vi "Is_TopLevel.vi"(8 "error in (no error)":errorcluster, 11 "AB_Source_RESTfulVI in":refnum<class "AB_Source_RESTfulVI.lvclass">) -> (0 "error out":errorcluster, 1 "openVIreference":bool, 2 "path":path, 3 "AB_Source_RESTfulVI out":refnum<class "AB_Source_RESTfulVI.lvclass">, 5 "readLinker":bool)   [LabVIEW 2020, in "AB_Source_RESTfulVI.lvclass"]
uses:
  <vilib>/AppBuilder/AB_Classes/Source/RESTfulVI/AB_Source_RESTfulVI.lvclass
  e:/builds/penguin/labview/branches/2020/dev/dist/vi.lib/AppBuilder/AB_Classes/Source/AB_Source.lvclass
  e:/builds/penguin/labview/branches/2020/dev/dist/vi.lib/AppBuilder/AB_Classes/Source/VI/AB_Source_VI.lvclass
  <resource>/Framework/Providers/Common/provcom_StringGlobals.vi
  <vilib>/AppBuilder/AB_Classes/Source/VI/AB_Source_VI.lvclass
  <vilib>/AppBuilder/AB_Classes/Source/AB_Source.lvclass
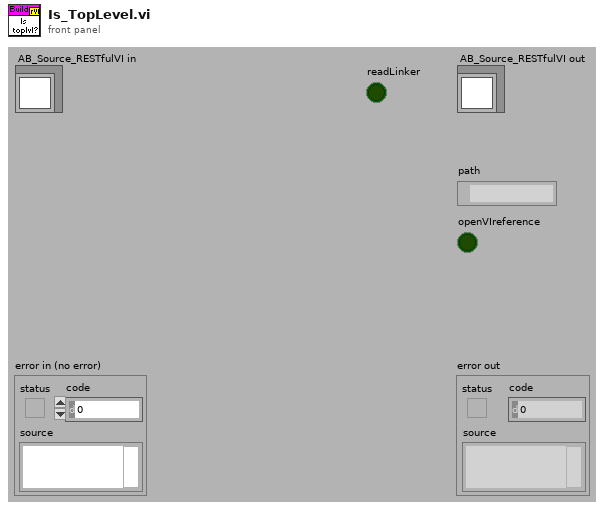
[diagram p1: front panel]
types:
  T1 = typedef "AB_Source.ctl" = cluster{"path":path, "itemID":string, "parentIndex":i32, "sourceInclusion":T2, "destinationIndex":i32, "properties":T3[], "newName":string, "lvfile":bool, "valid":bool, "eng_inBuild":bool, "eng_isNonVILink":bool, "Amalgamation":bool, "Amalgamation Piece":bool, "eng_delimitedName":string, "preventRename":bool}
  T2 = typedef "AB_Source_Inclusion.ctl" = enum16{"IncludeIfReferenced", "Include", "Exclude", "TopLevel"}
  T3 = typedef "AB_Source_Properties.ctl" = cluster{"sourcePropertyType":T4, "value":variant}
  T4 = typedef "AB_Source_Property_Type.ctl" = enum16{"Remove block diagram", "Remove front panel", "Password", "Window has title bar", "Show menu bar", "Show vertical scroll bar", "Show horizontal scroll bar", "Show toolbar", "Show Abort button", "Show fp when called", "Window behavior", "Allow user to close window", "Window run-time position", "Run when opened", "Allow debugging", "Auto error handling", "Generate guard code", "Use stack variables", "Expression folding", "Integer only", "Inline subVI"}
  T5 = typedef "AB_Source_VI.ctl" = cluster{"standardVI":bool, "dynamicDispatch":bool, "LLBtopLevel":bool, "privateDataControl":bool, "eng_hasNonVILinks":bool, "eng_reference":refnum<vi>, "eng_saveLevel":u32}
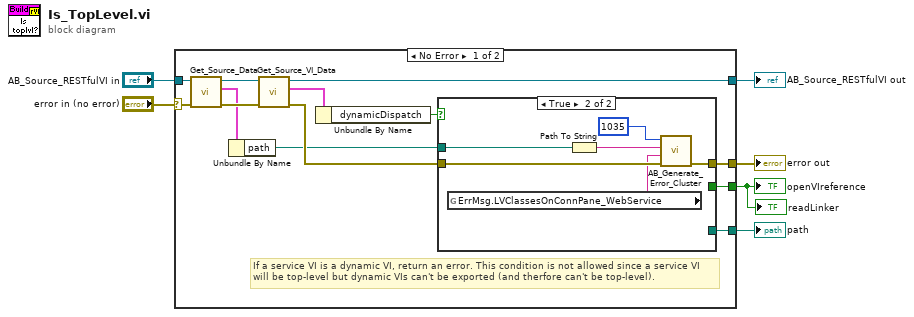
[diagram p0: block diagram]
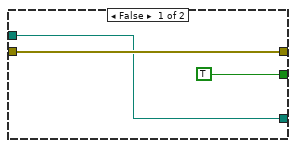
[diagram p2: hidden frame]
diagram:
  n1 = case shown="No Error" "error in (no error)" {
    selector: "error in (no error)" -> [w7 w29]
    tunnel: [w17 w30] -> w6
    tunnel: [w15 w29] -> w5
    tunnel: "AB_Source_RESTfulVI in" -> [w12 w30]
    tunnel: [w9 _] -> w3
    tunnel: [w8 _] -> w2
    frame No Error {
      # "If a service VI is a dynamic VI, return an error. This condition is not allowed since a service VI will be top-level but dynamic VIs can't be exported (and therfore can't be top-level)."
      n2 = call <vilib>:"Get_Source_Data.vi"("error in (no error)"=w7, "Class in"=w12) -> ("error out"=w13:errorcluster, "data"=w11:T1, "Class out"=w14:refnum<class "AB_Source_RESTfulVI.lvclass">)  [unwired: 7 out]
      n3 = Unbundle By Name(w11) -> ("path"=w10:path)
      n4 = call <vilib>:"Get_Source_VI_Data.vi"("error in (no error)"=w13, "Class in"=w14) -> ("error out"=w16:errorcluster, "data"=w19:T5, "Class out"=w17:refnum<class "AB_Source_RESTfulVI.lvclass">)  [unwired: 7 out]
      n5 = Unbundle By Name(w19) -> ("dynamicDispatch"=w18:bool)
      n6 = case shown="True" w18 {
        tunnel: w16 -> [w22 w25]
        tunnel: [w22 w24] -> w15
        tunnel: w10 -> [w21 w26]
        tunnel: [w21 _] -> w9
        tunnel: [TRUE _] -> w8
        frame False {
        }
        frame True {
          n7 = global read "provcom_StringGlobals.vi" "ErrMsg.LVClassesOnConnPane_WebService"() -> (w23:string)
          n8 = Path To String(path=w26) -> (string=w27:string)
          n9 = call <vilib>:"AB_Generate_Error_Cluster.vi"("error in (no error)"=w25, "Additional Message"=w23, "source"=w27, "Code"=1035 ("code")) -> ("error out"=w24:errorcluster)  [unwired: 7 out]
        }
      }
    }
    frame Error {
    }
  }
  "error out" <- w5
  "openVIreference" <- w2
  "path" <- w3
  "AB_Source_RESTfulVI out" <- w6
  "readLinker" <- w2
